vi "Write Log File.vi"(5 "Save Name":string="RAW-2048-0001-00400-002-400-", 7 "ROI Parameters":T1={"ROI (mm)"={"X (mm)"=1.0, "Y (mm)"=1.0}, "Shift (mm)"={"Xshift (mm)"=0.0, "Yshift (mm)"=0.0}}, 8 "Scan Parameter":string="2048(Pix-Camera)-2048 (#Z Op)-0001(#Arpt)-05 (ArptExtra)-00400(#A)-060(BrtnExtra)-002(#Brpt)-400(#B)", 9 "Aline Rate":u16(ring)=2 items=["76 KHz", "146 KHz", "76 KHz", "28 KHz", "10 KHz"], 10 "Objective":u16(ring) items=["5X LKM05", "10X LKM10", "20X LKM20", "10X LSM02"], 11 "Save Path":path=path "E:/Jiarui/1217test") -> ()   [LabVIEW 2017]
panel:
  in  "# Cscan":i32=1
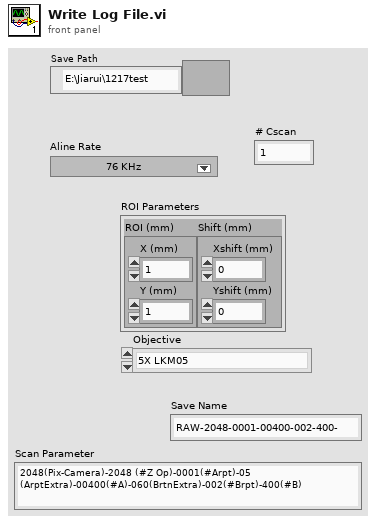
[diagram p1: front panel]
types:
  T1 = cluster{"ROI (mm)":cluster{"X (mm)":sgl, "Y (mm)":sgl}, "Shift (mm)":cluster{"Xshift (mm)":sgl, "Yshift (mm)":sgl}}
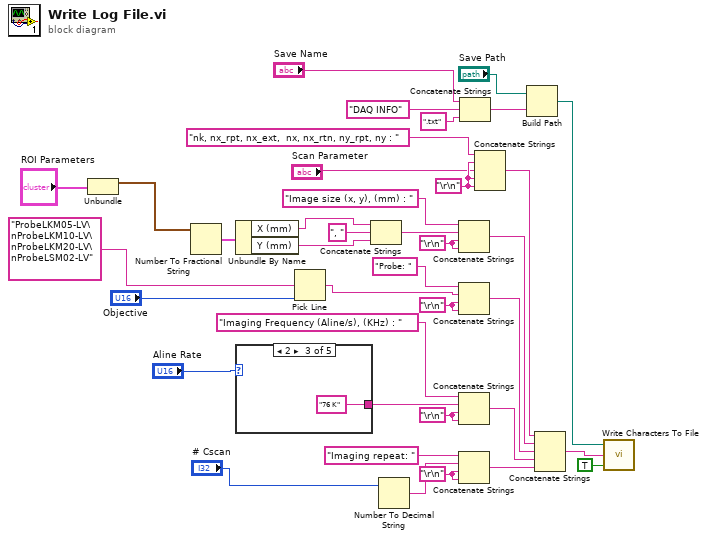
[diagram p0: block diagram]
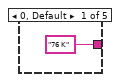
[diagram p2: hidden frame]
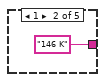
[diagram p3: hidden frame]
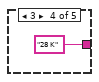
[diagram p4: hidden frame]
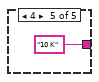
[diagram p5: hidden frame]
diagram:
  w16 = "\r\n"
  w20 = "\r\n"
  w28 = "\r\n"
  w29 = "\r\n"
  w12 = "\r\n"
  n1 = Unbundle("ROI Parameters") -> ("ROI (mm)"=w9:cluster{"X (mm)":sgl, "Y (mm)":sgl})  [unwired: 1 out]
  n2 = Number To Fractional String(number=w9) -> (F-format string=w11:cluster{"X (mm)":string, "Y (mm)":string})  [unwired: 3 in]
  n3 = Unbundle By Name(w11) -> ("X (mm)"=w34:string, "Y (mm)"=w35:string)
  n4 = case shown="2" "Aline Rate" {
    tunnel: ["76 K" "146 K" "76 K" "28 K" "10 K"] -> w15
    frame 0, Default {
    }
    frame 1 {
    }
    frame 2 {
    }
    frame 3 {
    }
    frame 4 {
    }
  }
  n5 = Pick Line(multi-line string="ProbeLKM05-LV\nProbeLKM10-LV\nProbeLKM20-LV\nProbeLSM02-LV" ("string (\"\")"), line index="Objective") -> (output string=w4:string)  [unwired: 1 in]
  n6 = Concatenate Strings(w34, ", " ("string"), w35) -> (w36:string)
  n7 = Number To Decimal String(number="# Cscan") -> (decimal integer string=w30:string)  [unwired: 1 in]
  n8 = Concatenate Strings("Image size (x, y), (mm) : " ("string"), w36, w29, w29) -> (w26:string)
  n9 = Concatenate Strings("Probe: " ("string"), w4, w20, w20) -> (w18:string)
  n10 = Concatenate Strings("Imaging Frequency (Aline/s), (KHz) : " ("string"), w15, w16, w16) -> (w13:string)
  n11 = Concatenate Strings("Imaging repeat: " ("string"), w30, w28, w28) -> (w17:string)
  n12 = Concatenate Strings("Save Name", "DAQ INFO" ("string"), ".txt" ("string")) -> (w38:string)
  n13 = Concatenate Strings("nk, nx_rpt, nx_ext,  nx, nx_rtn, ny_rpt, ny : " ("string"), w12, "Scan Parameter", w12, w12) -> (w27:string)
  n14 = Build Path(base path="Save Path", name or relative path=w38) -> (appended path=w24:path)
  n15 = Concatenate Strings(w27, w26, w18, w13, w17) -> (w25:string)
  n16 = call <vilib>:"Write Characters To File.vi"("append to file? (new file:F)"=TRUE, "character string"=w25, "file path (dialog if empty)"=w24) -> ()  [unwired: 2 in, 1 out]
